vi "Dummy Read Attributes.vi"(11 "Abstract Message Template in":refnum<class "Abstract Message Template.lvclass">) -> (2 "Payload":cluster{}, 3 "Abstract Message Template out":refnum<class "Abstract Message Template.lvclass">)   [LabVIEW 2020]
uses:
  Abstract Message Template/Abstract Message Template.lvclass
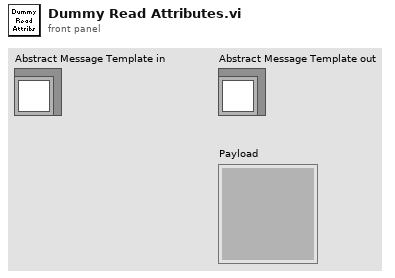
[diagram p1: front panel]
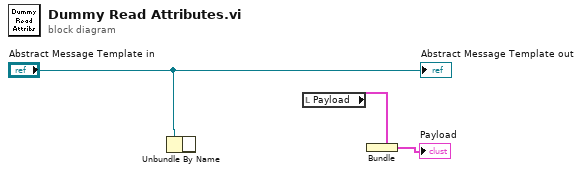
[diagram p0: block diagram]
diagram:
  n1 = Unbundle By Name("Abstract Message Template in") -> ()  [unwired: 1 out]
  n2 = local read "Payload"() -> (w1:cluster{})
  n3 = Bundle(cluster=w1) -> (→"Payload":cluster{"Boolean":void})  [unwired: 1 in]
  "Abstract Message Template out" <- "Abstract Message Template in"
